vi "_save_csv_CLC_Gen3_L1_GPS_ENA.vi"(5 "Marker_array":dbl[](array[numeric]), 7 "NoteName":string="SingleCh_", 11 "array in":string[][](array[string])) -> (3 "FileName":string)   [LabVIEW 2023]
uses:
  <vilib>/Utility/file.llb/Write Delimited Spreadsheet (string).vi
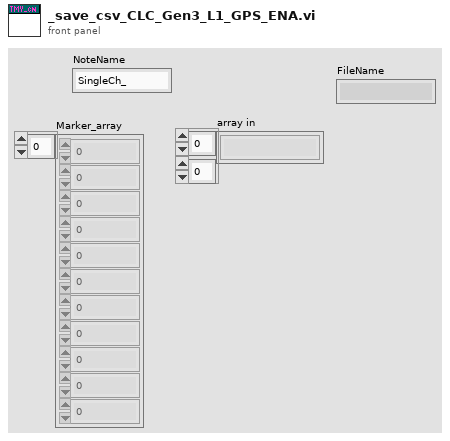
[diagram p1: front panel]
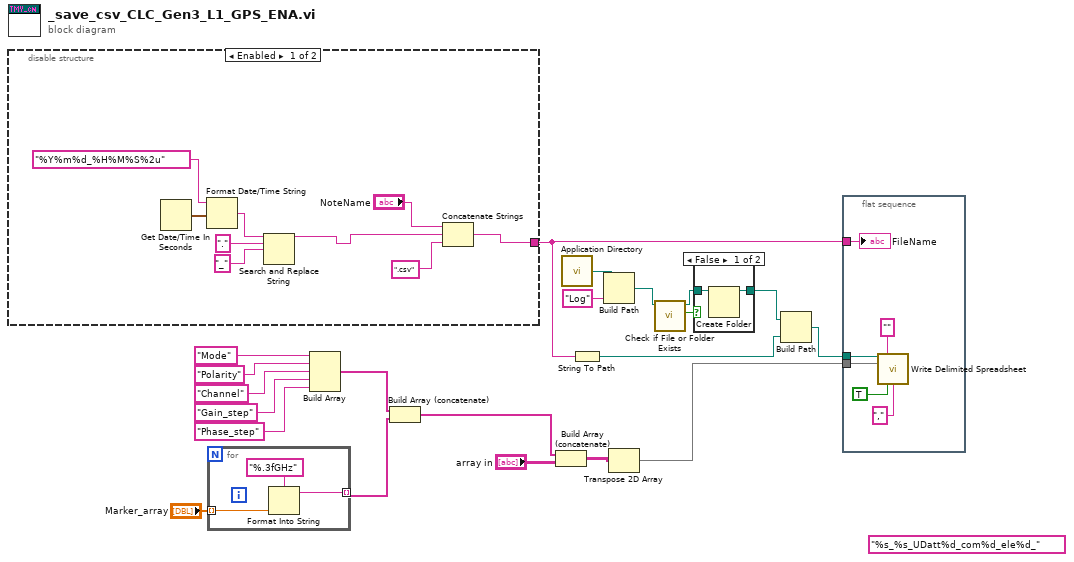
[diagram p0: block diagram]
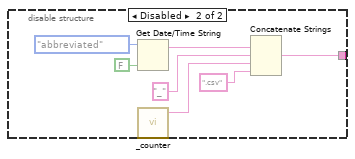
[diagram p3: hidden frame]
diagram:
  (unwired) "%s_%s_UDatt%d_com%d_ele%d_" ("format string")
  n1 = disable-structure shown="Enabled" {
    disable-tunnel: [w29 w31] -> w18
    frame Enabled {
      n2 = Get Date/Time In Seconds() -> (seconds since 1Jan1904=w27:timestamp)
      n3 = Format Date/Time String(time format string (%c)="%Y%m%d_%H%M%S%2u", seconds (now)=w27) -> (date/time string=w25:string)  [unwired: 1 in]
      n4 = Search and Replace String(input string=w25, search string=".", replace string="_") -> (result string=w22:string)  [unwired: 5 in, 3 out]
      n5 = Concatenate Strings("NoteName", w22, ".csv" ("delimiter (\\t)")) -> (w29:string)
    }
    frame Disabled {
      n6 = Get Date/Time String(date format (0)=enum16{"short", "long", "abbreviated"}."abbreviated", want seconds? (F)=FALSE) -> (date string=w38:string)  [unwired: 1 in, 1 out]
      n7 = call "_counter.vi"() -> ("out_count"=w32:string)  [unwired: 5 in]
      n8 = Concatenate Strings(w38, "_" ("delimiter (\\t)"), w32, ".csv" ("delimiter (\\t)")) -> (w31:string, w33:string)
    }
  }
  n9 = for {
    tunnel: "Marker_array" -> [w41] mode=indexing
    tunnel: [w39] -> w2 mode=indexing
    n10 = Format Into String(format string="%.3fGHz", w41) -> (resulting string=w39:string)  [unwired: 2 in, 1 out]
  }
  n11 = Build Array("Mode", "Polarity", "Channel", "Gain_step", "Phase_step") -> (w3:string[])
  n12 = Build Array (concatenate)(w3, w2) -> (w1:string[])
  n13 = Build Array (concatenate)(w1, "array in") -> (w10:string[][])
  n14 = call <vilib>:"Application Directory.vi"() -> ("Application Directory"=w17:path)
  n15 = String To Path(string=w18) -> (path=w20:path)
  n16 = Build Path(base path=w17, name or relative path="Log") -> (appended path=w14:path)
  n17 = Transpose 2D Array(2D array=w10) -> (transposed array=w12:string[][])
  n18 = call <vilib>:"Check if File or Folder Exists.vi"("path"=w14) -> ("file or folder exists?"=w16:bool, "dup path"=w15:path)  [unwired: 8 in, 1 out]
  n19 = case shown="False" w16 {
    tunnel: w15 -> [w43 w44]
    tunnel: [w42 w44] -> w13
    frame False {
      n20 = Create Folder(path (use dialog)=w43) -> (created path=w42:path)  [unwired: 2 in, 2 out]
    }
    frame True {
    }
  }
  n21 = Build Path(base path=w13, name or relative path=w20) -> (appended path=w19:path)
  n22 = flat-sequence {
    tunnel: w19 -> [w49]
    tunnel: w18 -> [w47]
    tunnel: w12 -> [w45]
    frame #0 {
      n23 = call-poly <vilib>:"Write Delimited Spreadsheet.vi"("file path (dialog if empty)"=w49, "format (%s)"="" ("format (%.3f)"), "2D data"=w45, "transpose? (no:F)"=TRUE, "delimiter (\\t)"="," ("delimiter (\\t)")) -> ()  [unwired: 9 in, 2 out]
      "FileName" <- w47
    }
  }
